vi "Misc Ignore Timeout Error.vi"(8 "error in (no error)":errorcluster) -> (0 "error out":errorcluster)   [LabVIEW 2011, in "Misc VIs.lvlib"]
uses:
  Misc VIs.lvlib
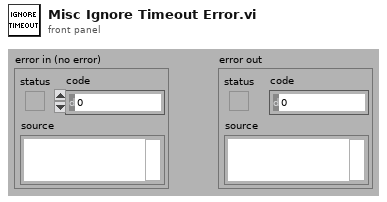
[diagram p1: front panel]
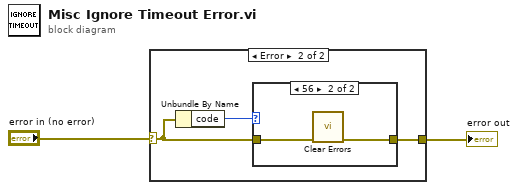
[diagram p0: block diagram]
diagram:
  n1 = case shown="Error" "error in (no error)" {
    selector: "error in (no error)" -> [w3 w5]
    tunnel: [w3 w4] -> w1
    frame No Error {
    }
    frame Error {
      n2 = Unbundle By Name(w5) -> ("code"=w6:i32)
      n3 = case shown="56" w6 {
        tunnel: w5 -> [w7 w9]
        tunnel: [w7 w8] -> w4
        frame 0, Default {
        }
        frame 56 {
          n4 = call <vilib>:"Clear Errors.vi"("error in (no error)"=w9) -> ("error out"=w8:errorcluster)  [unwired: 6 out]
        }
      }
    }
  }
  "error out" <- w1
